vi "String conversion %LF.vi"(7 "Conversion":enum16{"LF à %LF", "%LF à LF"}(ring), 11 "String IN":string) -> (3 "String OUT":string)   [LabVIEW 2013]
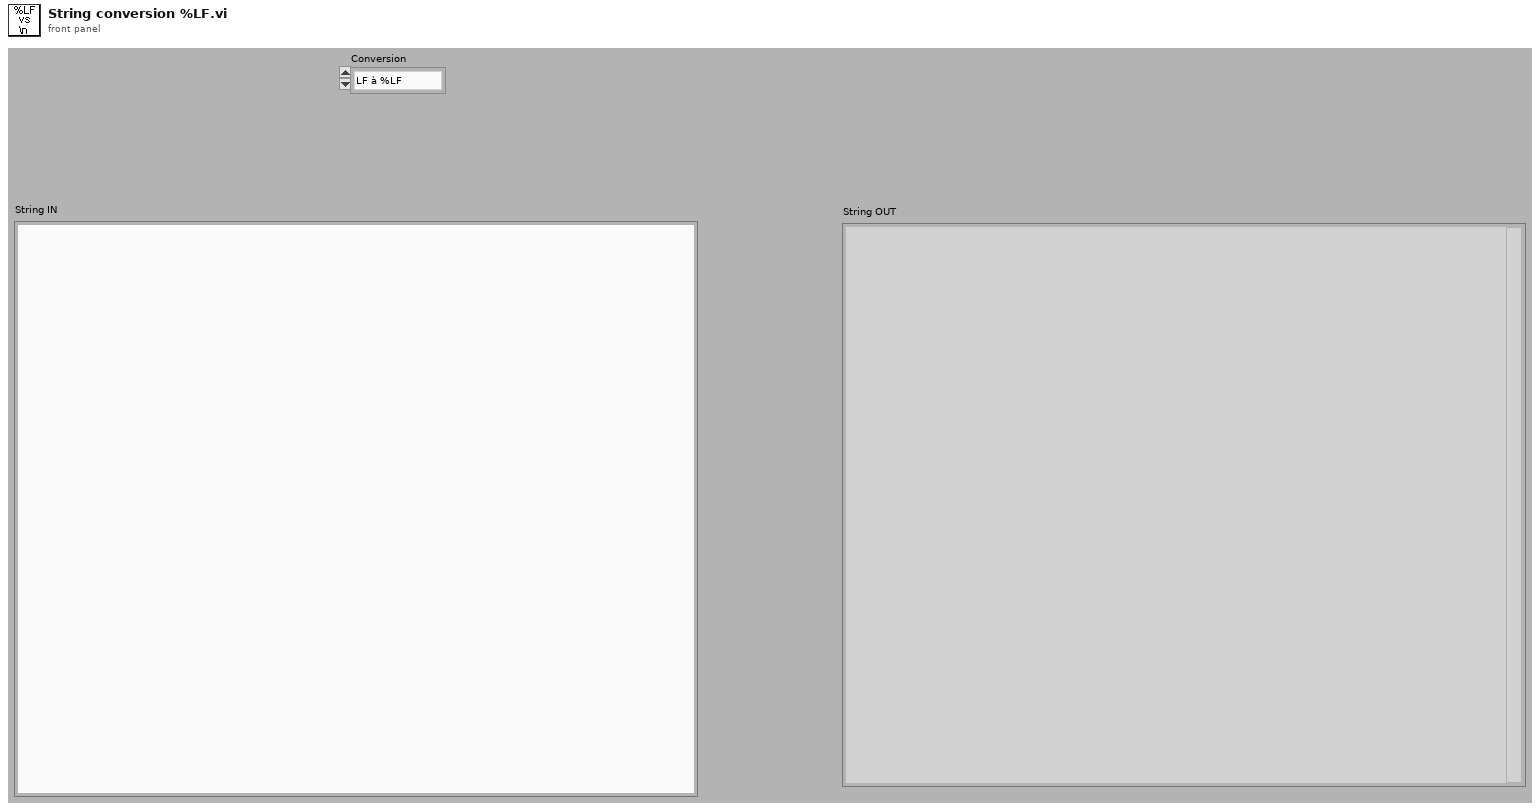
[diagram p1: front panel]
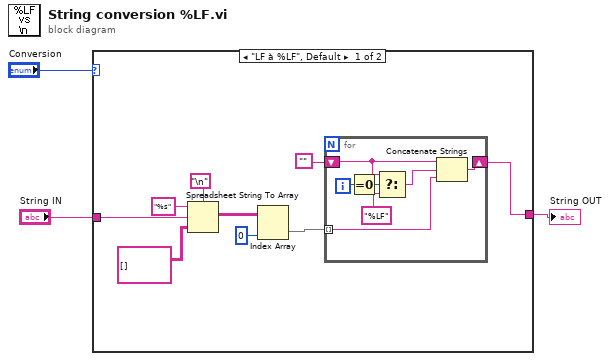
[diagram p0: block diagram]
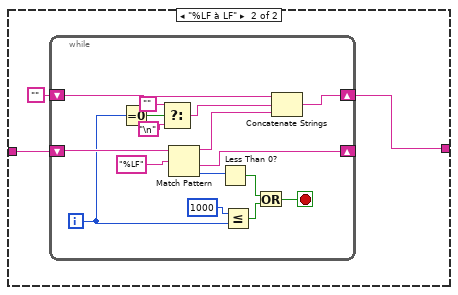
[diagram p2: hidden frame]
diagram:
  n1 = case shown="\"LF à %LF\", Default" "Conversion" {
    tunnel: "String IN" -> [w12 w22]
    tunnel: [w4 w20] -> w2
    frame "LF à %LF", Default {
      n2 = Spreadsheet String To Array(delimiter (Tab)="\n", format string="%s", spreadsheet string=w12, array type (2D Dbl)=string[][] []) -> (array=w8:string[][])
      n3 = Index Array(array=w8, index (col)=0 ("disabled index (col)")) -> (element=w6:string[])  [unwired: 1 in]
      n4 = for {
        tunnel: w6 -> [w19] mode=indexing
        shift-right: [w18] -> w4
        shift-left: "" -> [w15]
        i -> [w16]
        n5 = Equal To 0?(x=w16) -> (x = 0?=w17:bool)
        n6 = Select(t=w15, s=w17, f="%LF" ("string")) -> (s? t:f=w14:string)
        n7 = Concatenate Strings(w15, w14, w19) -> (w18:string)
      }
    }
    frame "%LF à LF" {
      n8 = while {
        shift-right: [w36] -> _
        shift-left: w22 -> [w38]
        shift-right: [w32] -> w20
        shift-left: "" -> [w35]
        i -> [w26]
        stop <- w28 stop-if-true
        n9 = Equal To 0?(x=w26) -> (x = 0?=w27:bool)
        n10 = Select(t="", s=w27, f="\n") -> (s? t:f=w23:string)
        n11 = Match Pattern(string=w38, regular expression="%LF" ("string")) -> (before substring=w34:string, after substring=w36:string, offset past match=w33:i32)  [unwired: 2 out]
        n12 = Less Than 0?(x=w33) -> (x < 0?=w30:bool)
        n13 = Less Or Equal?(x=1000, y=w26) -> (x <= y?=w29:bool)
        n14 = Or(x=w30, y=w29) -> (x .or. y?=w28:bool)
        n15 = Concatenate Strings(w35, w23, w34) -> (w32:string)
      }
    }
  }
  "String OUT" <- w2
